vi "Global temperature.vi"() -> ()   [LabVIEW 2023]
panel:
  in  "Temperature":dbl
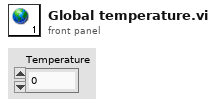
[diagram p1: front panel]
diagram:
